vi "在线监测仪器仪表参数.vi"() -> ()   [LabVIEW 2016, in "MB SLAVE.lvlib"]
uses:
  MB SLAVE.lvlib
panel:
  in  "浊度参数":T1={"测量量程"=0.0, "测量精度"=0.0, "测量间隔"=0.0, "消解温度"=0.0, "消解时长"=0.0, "空白校准时间"=timestamp(0 s since 1904-01-01), "曲线截距"=0.0, "曲线斜率"=0.0, "测量检出限"=0.0, "测量信号值"=0.0, "线性相关系数"=0.0, "二次多项式系数"=0.0, "标样校准时间"=timestamp(0 s since 1904-01-01), "单位"=enum."mg/L"}
  in  "电导率参数":T1={"测量量程"=0.0, "测量精度"=0.0, "测量间隔"=0.0, "消解温度"=0.0, "消解时长"=0.0, "空白校准时间"=timestamp(0 s since 1904-01-01), "曲线截距"=0.0, "曲线斜率"=0.0, "测量检出限"=0.0, "测量信号值"=0.0, "线性相关系数"=0.0, "二次多项式系数"=0.0, "标样校准时间"=timestamp(0 s since 1904-01-01), "单位"=enum."mg/L"}
  in  "溶解氧参数":T1={"测量量程"=0.0, "测量精度"=0.0, "测量间隔"=0.0, "消解温度"=0.0, "消解时长"=0.0, "空白校准时间"=timestamp(0 s since 1904-01-01), "曲线截距"=0.0, "曲线斜率"=0.0, "测量检出限"=0.0, "测量信号值"=0.0, "线性相关系数"=0.0, "二次多项式系数"=0.0, "标样校准时间"=timestamp(0 s since 1904-01-01), "单位"=enum."mg/L"}
  in  "PH参数":T1={"测量量程"=0.0, "测量精度"=0.0, "测量间隔"=0.0, "消解温度"=0.0, "消解时长"=0.0, "空白校准时间"=timestamp(0 s since 1904-01-01), "曲线截距"=0.0, "曲线斜率"=0.0, "测量检出限"=0.0, "测量信号值"=0.0, "线性相关系数"=0.0, "二次多项式系数"=0.0, "标样校准时间"=timestamp(0 s since 1904-01-01), "单位"=enum."mg/L"}
  in  "水温参数":T1={"测量量程"=0.0, "测量精度"=0.0, "测量间隔"=0.0, "消解温度"=0.0, "消解时长"=0.0, "空白校准时间"=timestamp(0 s since 1904-01-01), "曲线截距"=0.0, "曲线斜率"=0.0, "测量检出限"=0.0, "测量信号值"=0.0, "线性相关系数"=0.0, "二次多项式系数"=0.0, "标样校准时间"=timestamp(0 s since 1904-01-01), "单位"=enum."mg/L"}
  in  "CODCr参数":T1={"测量量程"=0.0, "测量精度"=0.0, "测量间隔"=0.0, "消解温度"=0.0, "消解时长"=0.0, "空白校准时间"=timestamp(0 s since 1904-01-01), "曲线截距"=0.0, "曲线斜率"=0.0, "测量检出限"=0.0, "测量信号值"=0.0, "线性相关系数"=0.0, "二次多项式系数"=0.0, "标样校准时间"=timestamp(0 s since 1904-01-01), "单位"=enum."mg/L"}
  in  "总氮参数":T1={"测量量程"=0.0, "测量精度"=0.0, "测量间隔"=0.0, "消解温度"=0.0, "消解时长"=0.0, "空白校准时间"=timestamp(0 s since 1904-01-01), "曲线截距"=0.0, "曲线斜率"=0.0, "测量检出限"=0.0, "测量信号值"=0.0, "线性相关系数"=0.0, "二次多项式系数"=0.0, "标样校准时间"=timestamp(0 s since 1904-01-01), "单位"=enum."mg/L"}
  in  "总磷参数":T1={"测量量程"=0.0, "测量精度"=0.0, "测量间隔"=0.0, "消解温度"=0.0, "消解时长"=0.0, "空白校准时间"=timestamp(0 s since 1904-01-01), "曲线截距"=0.0, "曲线斜率"=0.0, "测量检出限"=0.0, "测量信号值"=0.0, "线性相关系数"=0.0, "二次多项式系数"=0.0, "标样校准时间"=timestamp(0 s since 1904-01-01), "单位"=enum."mg/L"}
  in  "氨氮参数":T1={"测量量程"=0.0, "测量精度"=0.0, "测量间隔"=0.0, "消解温度"=0.0, "消解时长"=0.0, "空白校准时间"=timestamp(0 s since 1904-01-01), "曲线截距"=0.0, "曲线斜率"=0.0, "测量检出限"=0.0, "测量信号值"=0.0, "线性相关系数"=0.0, "二次多项式系数"=0.0, "标样校准时间"=timestamp(0 s since 1904-01-01), "单位"=enum."mg/L"}
  in  "CODMn参数":T1={"测量量程"=0.0, "测量精度"=0.0, "测量间隔"=0.0, "消解温度"=0.0, "消解时长"=0.0, "空白校准时间"=timestamp(0 s since 1904-01-01), "曲线截距"=0.0, "曲线斜率"=0.0, "测量检出限"=0.0, "测量信号值"=0.0, "线性相关系数"=0.0, "二次多项式系数"=0.0, "标样校准时间"=timestamp(0 s since 1904-01-01), "单位"=enum."mg/L"}
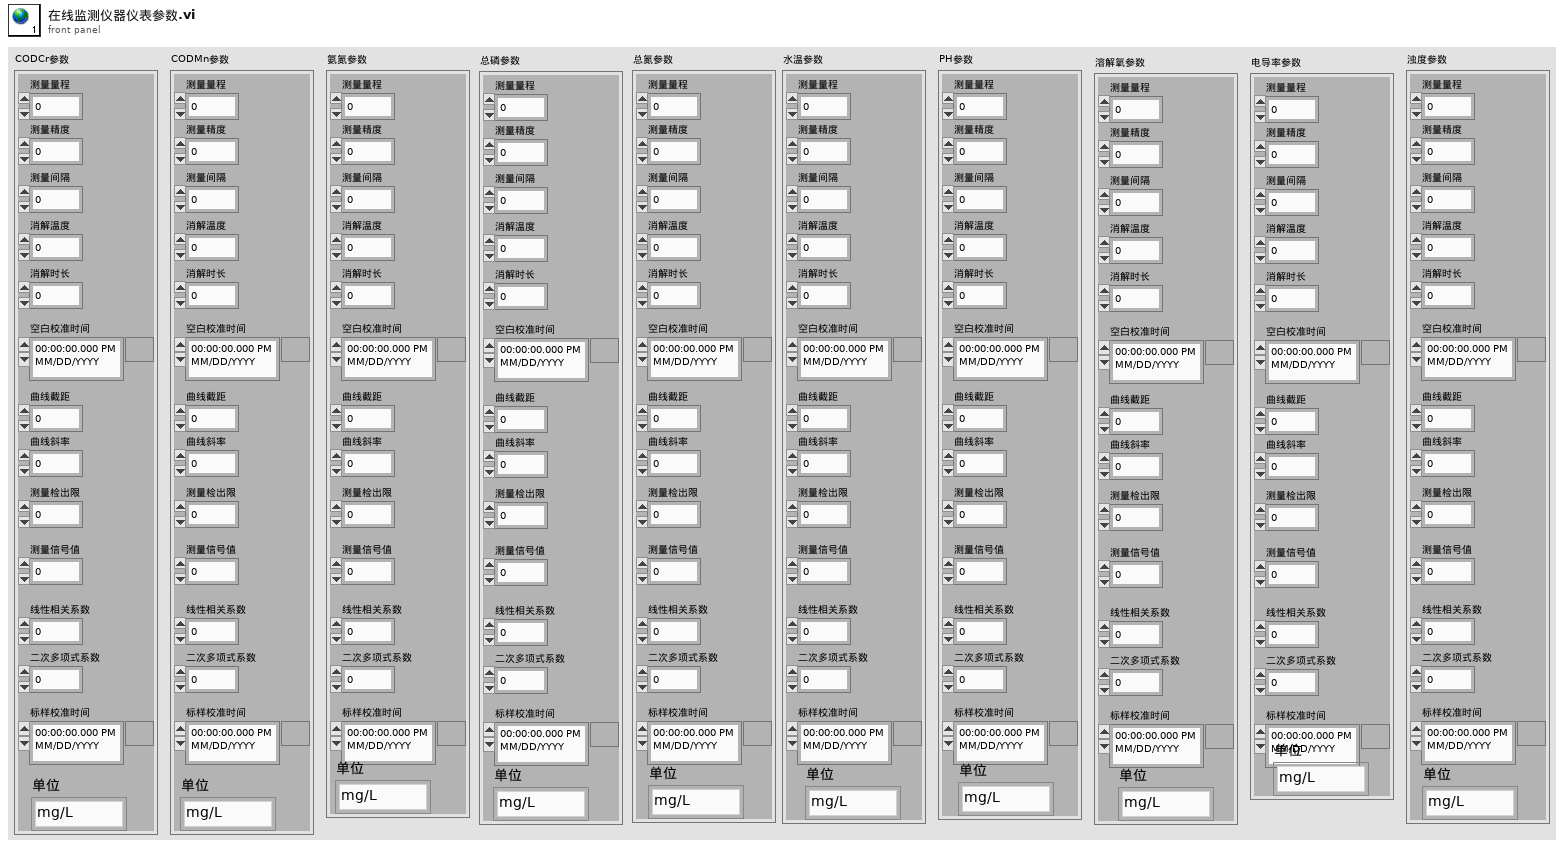
[diagram p1: front panel]
types:
  T1 = cluster{"测量量程":dbl, "测量精度":dbl, "测量间隔":dbl, "消解温度":dbl, "消解时长":dbl, "空白校准时间":timestamp, "曲线截距":dbl, "曲线斜率":dbl, "测量检出限":dbl, "测量信号值":dbl, "线性相关系数":dbl, "二次多项式系数":dbl, "标样校准时间":timestamp, "单位":enum16{"ug/L", "mg/L"}}
diagram:
